vi "AddDependency.vi"(8 "error in (no error)":errorcluster, 9 "Level":string, 10 "Dependency":refnum<class "SMO.lvclass">, 11 "SMO in":refnum<class "SMO.lvclass">) -> (0 "error out":errorcluster, 3 "SMO out":refnum<class "SMO.lvclass">)   [LabVIEW 2013, in "SMO.lvclass"]
uses:
  SMO.lvclass
  Typedefs/SMO Dependency--Cluster.ctl
  SMO.lvclass/SMO.ctl
  <vilib>/regexp/Match Regular Expression.xnode
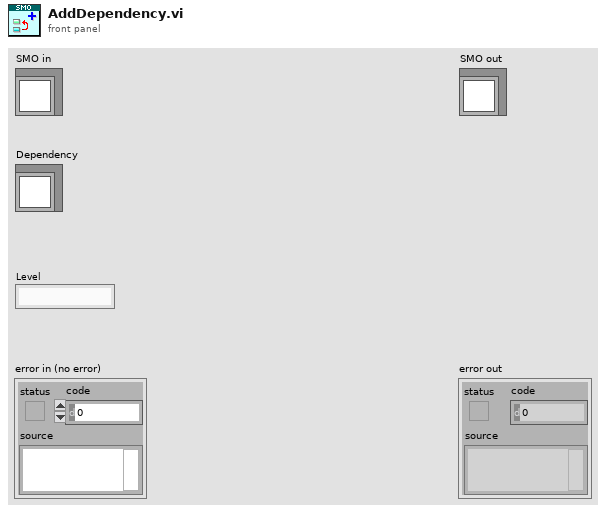
[diagram p1: front panel]
types:
  T1 = typedef "SMO.lvclass/SMO Dependency--Cluster.ctl" = cluster{"Dependency":refnum<class "SMO.lvclass">, "Level":string}
  T2 = typedef "SMO.lvclass/PrivateData--Ref.ctl" = refnum<data-value>
  T3 = typedef "SMO.lvclass/PrivateData--Cluster.ctl" = cluster{"Parent Call":T4, "Registered Processes":T5[], "Sync Notifier":refnum<notifier>, "Process Error Notifier":refnum<notifier>, "Protected Events":T6, "Public Events":T7, "SMO State":T8, "[Dependencies]":T1[], "[Attributes]":refnum<class "Attribute.lvclass">[], "Launcher Close":refnum<notifier>}
  T4 = typedef "SMO.lvclass/Parent Call--Enum.ctl" = enum16{"Allows parent to run", "Does not request parent to run"}
  T5 = typedef "SMO.lvclass/RegisteredProcessData--Cluster.ctl" = cluster{"Name":string, "Static VI Ref":refnum<vi>, "Running":bool, "NotifierRef":u32}
  T6 = typedef "SMO.lvclass/Protected Events.ctl" = cluster{"StopProcesses":refnum<user-event>, "AbortProcesses":refnum<user-event>, "Config Changed":refnum<user-event>}
  T7 = typedef "SMO.lvclass/Public Events.ctl" = cluster{"Error":refnum<user-event>, "State":refnum<user-event>}
  T8 = typedef "SMO.lvclass/SMOState --Enum.ctl" = enum16{"unknown", "Created", "Started", "Stopped"}
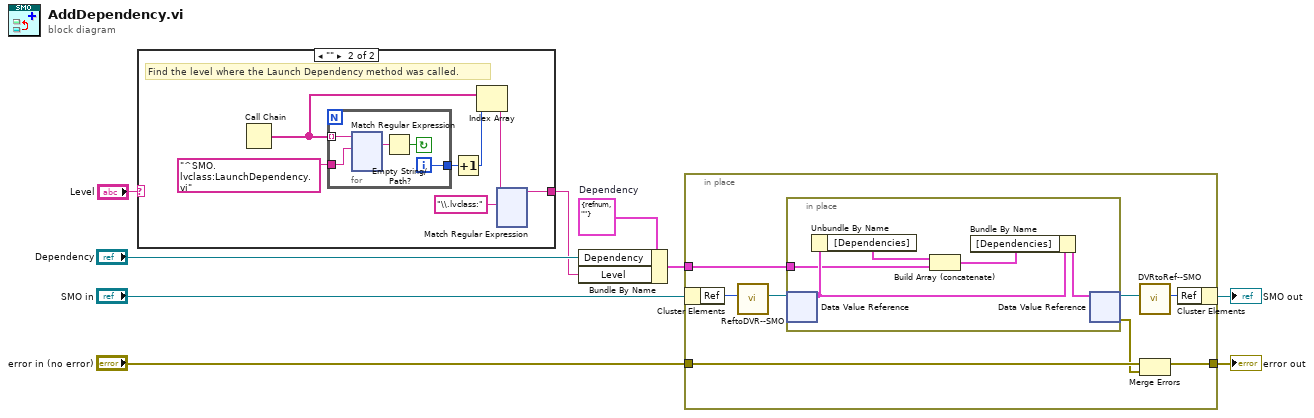
[diagram p0: block diagram]
diagram:
  w7 = T1 {"Dependency"=refnum, "Level"=""}  # Dependency
  n1 = case shown="\"\"" "Level" {
    selector: "Level" -> [w10 _]
    tunnel: [w10 w11] -> w2
    frame Default {
    }
    frame "" {
      # "Find the level where the Launch Dependency method was called."
      n2 = Call Chain() -> (call chain=w16:string[])
      n3 = for {
        tunnel: w16 -> [w136] mode=indexing
        tunnel: "^SMO.lvclass:LaunchDependency.vi" -> [w135]
        tunnel: [w132] -> w15
        i -> [w132]
        stop <- w133 continue-if-true
        n4 = xnode "Match Regular Expression"("input string"=w136, "regular expression"=w135) -> ("whole match"=w134:string)  [unwired: 4 in, 4 out]
        n5 = Empty String/Path?(string/path=w134) -> (empty?=w133:bool)
      }
      n6 = Increment(x=w15) -> (x+1=w14:i32)
      n7 = Index Array(array=w16, index=w14) -> (element=w13:string)
      n8 = xnode "Match Regular Expression"("input string"=w13, "regular expression"="\\.lvclass:") -> ("before match"=w11:string)  [unwired: 4 in, 4 out]
    }
  }
  n9 = Bundle By Name(cluster=w7, "Dependency"="Dependency", "Level"=w2) -> (w5:T1)
  n10 = in-place {
    in-place-border: "error in (no error)" -> [w254]
    in-place-border: [w252] -> w8
    in-place-border: w5 -> [w251]
    n11 = in-place-cluster #1("SMO in") -> ("Ref"=w258:u32)
    n12 = call "ReftoDVR--SMO.vi"("Ref"=w258) -> ("Ref"=w257:T2)  [unwired: 10 in]
    n13 = in-place {
      in-place-border: w251 -> [w260]
      n14 = in-place-dvr #2(w257) -> (w262:T3)  [unwired: 1 out]
      n15 = Unbundle By Name(w262) -> ("[Dependencies]"=w261:T1[])
      n16 = Build Array (concatenate)(w261, w260) -> (w259:T1[])
      n17 = Bundle By Name(cluster=w262, "[Dependencies]"=w259) -> (w263:T3)
      n18 = in-place-dvr #2(w263) -> (w256:T2, w253:errorcluster)
    }
    n19 = call "DVRtoRef--SMO.vi"("Ref"=w256) -> ("Ref"=w255:u32)  [unwired: 10 in]
    n20 = Merge Errors(w254, w253) -> (w252:errorcluster)
    n21 = in-place-cluster #1("Ref"=w255) -> (→"SMO out":refnum<class "SMO.lvclass">)
  }
  "error out" <- w8
